vi "Adjust_VI_Properties.vi"(6 "VI refnum in":refnum<vi>, 8 "error in (no error)":errorcluster, 9 "sourceInclusion":T3, 10 "properties in":T1[](array[typedef]), 11 "AB_Targetfile in":refnum<class "AB_Targetfile.lvclass">) -> (0 "error out":errorcluster, 1 "defaultSaveLevel":u32, 2 "properties out":T1[](array[typedef]), 3 "AB_Targetfile out":refnum<class "AB_Targetfile.lvclass">)   [LabVIEW 2020, in "AB_Targetfile.lvclass"]
uses:
  <vilib>/AppBuilder/AB_Classes/TargetFile/AB_Targetfile.lvclass
  <vilib>/AppBuilder/AB_Source_Properties.ctl
  <vilib>/AppBuilder/AB_Source_Property_Type.ctl
  <vilib>/AppBuilder/AB_Source_Inclusion.ctl
  <vilib>/AppBuilder/AB_Classes/TargetFile/AB_Targetfile.lvclass/AB_Targetfile.ctl
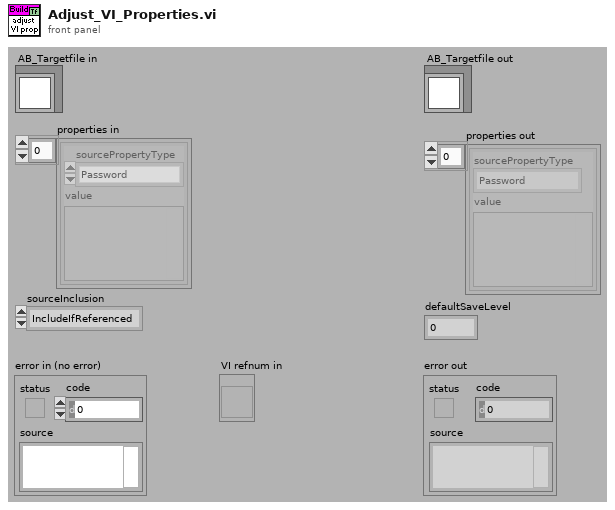
[diagram p1: front panel]
types:
  T1 = typedef "AB_Source_Properties.ctl" = cluster{"sourcePropertyType":T2, "value":variant}
  T2 = typedef "AB_Source_Property_Type.ctl" = enum16{"Remove block diagram", "Remove front panel", "Password", "Window has title bar", "Show menu bar", "Show vertical scroll bar", "Show horizontal scroll bar", "Show toolbar", "Show Abort button", "Show fp when called", "Window behavior", "Allow user to close window", "Window run-time position", "Run when opened", "Allow debugging", "Auto error handling", "Generate guard code", "Use stack variables", "Expression folding", "Integer only", "Inline subVI"}
  T3 = typedef "AB_Source_Inclusion.ctl" = enum16{"IncludeIfReferenced", "Include", "Exclude", "TopLevel"}
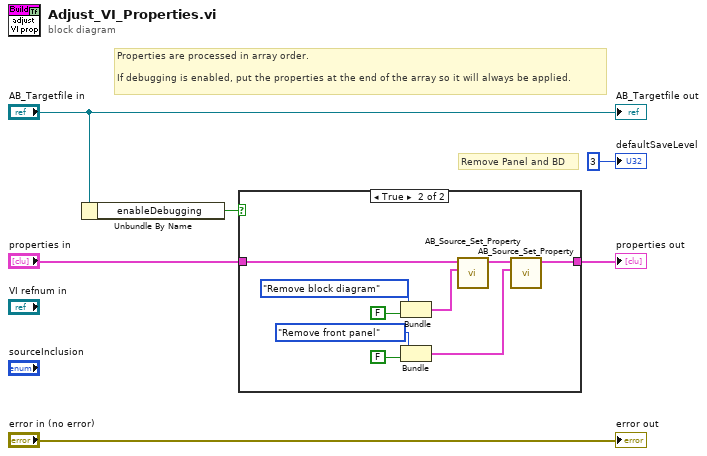
[diagram p0: block diagram]
diagram:
  # "Remove Panel and BD"
  # "Properties are processed in array order.\n\nIf debugging is enabled, put the properties at the end of the array so it will always be applied."
  n1 = Unbundle By Name("AB_Targetfile in") -> ("enableDebugging"=w5:bool)
  n2 = case shown="True" w5 {
    tunnel: "properties in" -> [w7 w12]
    tunnel: [w7 w10] -> w2
    frame False {
    }
    frame True {
      n3 = Bundle("sourcePropertyType"=AB_Source_Property_Type."Remove block diagram", FALSE) -> (w9:cluster{"sourcePropertyType":T2, bool})  [unwired: 1 out]
      n4 = Bundle("sourcePropertyType"=AB_Source_Property_Type."Remove front panel", FALSE) -> (w8:cluster{"sourcePropertyType":T2, bool})  [unwired: 1 out]
      n5 = call <vilib>:"AB_Source_Set_Property.vi"("sourceProperty"=w9, "sourceProperties in"=w12) -> ("sourceProperties out"=w11:T1[])  [unwired: 1 in, 8 out]
      n6 = call <vilib>:"AB_Source_Set_Property.vi"("sourceProperty"=w8, "sourceProperties in"=w11) -> ("sourceProperties out"=w10:T1[])  [unwired: 1 in, 8 out]
    }
  }
  "properties out" <- w2
  "error out" <- "error in (no error)"
  "defaultSaveLevel" <- u32 3 ("defaultSaveLevel")
  "AB_Targetfile out" <- "AB_Targetfile in"
